vi "SQL Data Filter.vi"(10 "SQL Reply Data":string[][](array[string])) -> (2 "appended array":cluster{timestamp[], dbl[]}[](array[cluster]))   [LabVIEW 2019]
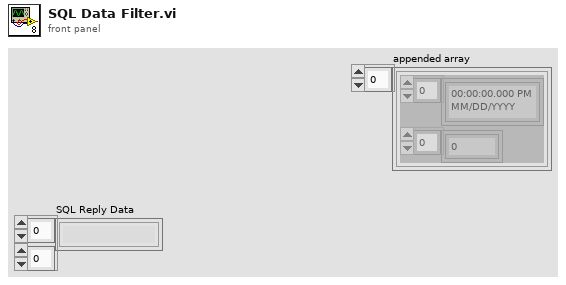
[diagram p1: front panel]
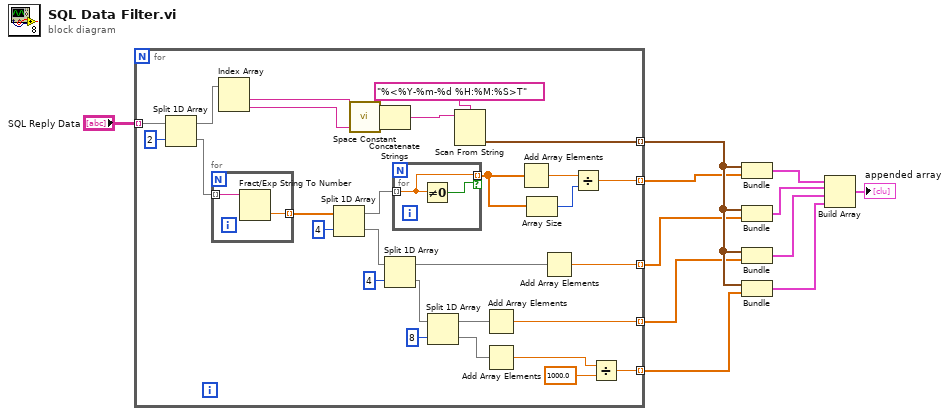
[diagram p0: block diagram]
diagram:
  n1 = for {
    tunnel: "SQL Reply Data" -> [w34] mode=indexing
    tunnel: [w37] -> w10 mode=indexing
    tunnel: [w36] -> w9 mode=indexing
    tunnel: [w14] -> w6 mode=indexing
    tunnel: [w13] -> w4 mode=indexing
    tunnel: [w22] -> w3 mode=indexing
    n2 = Split 1D Array(array=w34, index=2) -> (first subarray=w32:string[], second subarray=w29:string[])
    n3 = for {
      tunnel: w29 -> [w44] mode=indexing
      tunnel: [w43] -> w28 mode=indexing
      n4 = Fract/Exp String To Number(string=w44) -> (number=w43:dbl)  [unwired: 3 in, 1 out]
    }
    n5 = Index Array(array=w32) -> (element #1=w31:string, element #2=w30:string)  [unwired: 2 in]
    n6 = Split 1D Array(array=w28, index=4) -> (first subarray=w18:dbl[], second subarray=w19:dbl[])
    n7 = call <vilib>:"Space Constant.vi"() -> ("String"=w40:string)
    n8 = Concatenate Strings(w31, w40, w30) -> (w38:string)
    n9 = Split 1D Array(array=w19, index=4) -> (first subarray=w12:dbl[], second subarray=w25:dbl[])
    n10 = for {
      tunnel: w18 -> [w42] mode=indexing
      tunnel: [w42] -> w17 mode=indexing if=w41
      n11 = Not Equal To 0?(x=w42) -> (x != 0?=w41:bool)
    }
    n12 = Split 1D Array(array=w25, index=8) -> (first subarray=w23:dbl[], second subarray=w21:dbl[])
    n13 = Scan From String(format string="%<%Y-%m-%d %H:%M:%S>T", input string=w38) -> (output 1=w37:timestamp)  [unwired: 3 in, 3 out]
    n14 = Add Array Elements(numeric array=w23) -> (sum=w22:dbl)
    n15 = Add Array Elements(numeric array=w21) -> (sum=w20:dbl)
    n16 = Add Array Elements(numeric array=w17) -> (sum=w15:dbl)
    n17 = Array Size(array=w17) -> (size(s)=w16:i32)
    n18 = Add Array Elements(numeric array=w12) -> (sum=w13:dbl)
    n19 = Divide(x=w15, y=w16) -> (x/y=w14:dbl)
    n20 = Divide(x=w20, y=1000.0) -> (x/y=w36:dbl)
  }
  n21 = Bundle(w10, w6) -> (w5:cluster{timestamp[], dbl[]})  [unwired: 1 in]
  n22 = Bundle(w10, w4) -> (w2:cluster{timestamp[], dbl[]})  [unwired: 1 in]
  n23 = Bundle(w10, w3) -> (w1:cluster{timestamp[], dbl[]})  [unwired: 1 in]
  n24 = Bundle(w10, w9) -> (w8:cluster{timestamp[], dbl[]})  [unwired: 1 in]
  n25 = Build Array(w5, w2, w1, w8) -> (→"appended array":cluster{timestamp[], dbl[]}[])
